vi "IECal-Compute ASTF.vi"(0 "Stimulus":dbl[](array[numeric]), 5 "Response":dbl[](array[numeric]), 7 "Fs (Hz)":dbl, 9 "Response":T1, 11 "error in (no error)":errorcluster) -> (6 "data":T2, 15 "error out":errorcluster)   [LabVIEW 2020]
uses:
  Common VIs/Typedefs/CAL-Data.ctl
  Typedefs/IECal-Response.ctl
  epl-vi-lib/Utility VIs/Math VIs/FFT x(t) to dB,Degrees (1D).vi
panel:
  out "Frequency":dbl[](array[numeric])
  out "ASTF Phase":dbl[](array[numeric])
  out "ASTF Mag":dbl[](array[numeric])
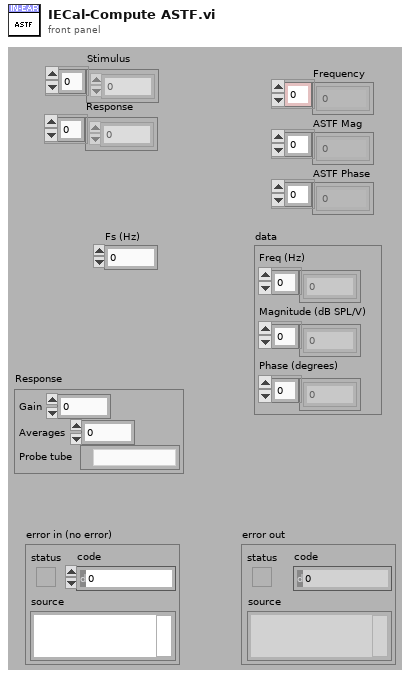
[diagram p1: front panel]
types:
  T1 = typedef "IECal-Response.ctl" = cluster{"Gain":dbl, "Averages":i32, "Probe tube":path}
  T2 = typedef "CAL-Data.ctl" = cluster{"Freq (Hz)":dbl[], "Magnitude (dB SPL/V)":dbl[], "Phase (degrees)":dbl[]}
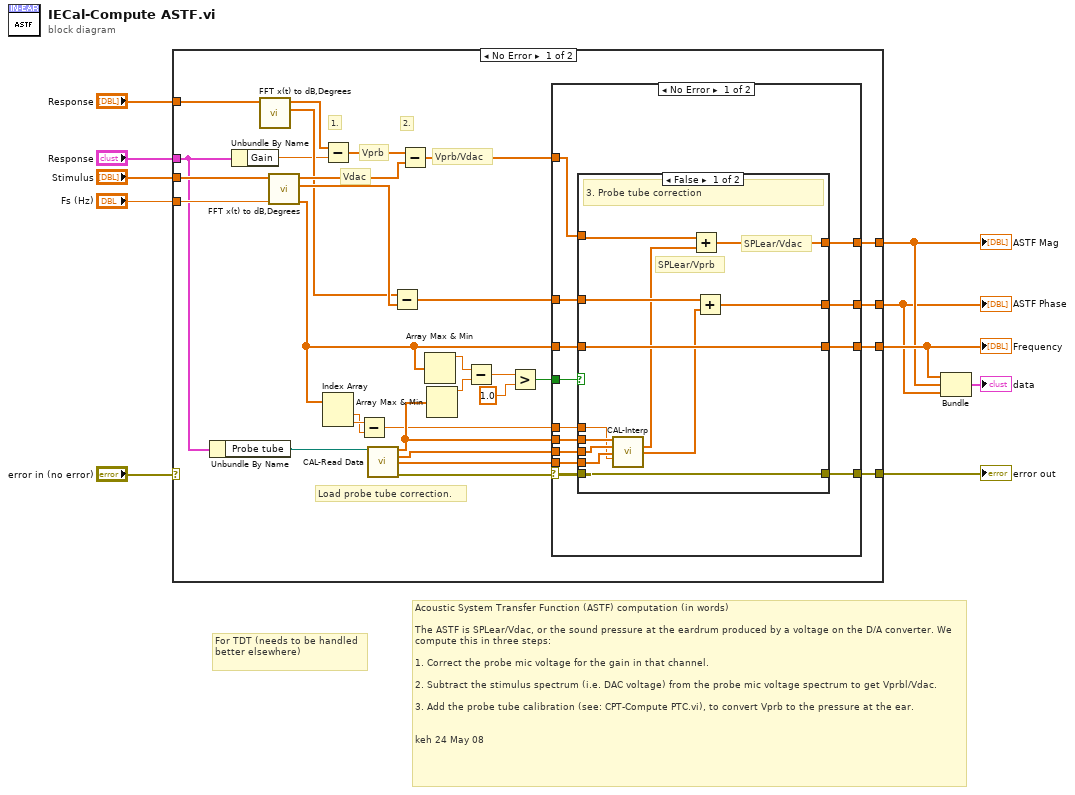
[diagram p0: block diagram]
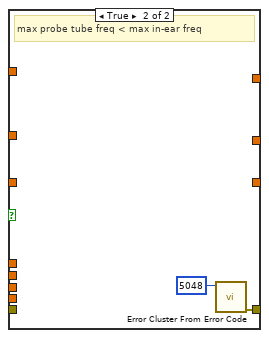
[diagram p2: hidden frame]
diagram:
  # "For TDT (needs to be handled better elsewhere)"
  # "Acoustic System Transfer Function (ASTF) computation (in words)\n\nThe ASTF is SPLear/Vdac, or the sound pressure at the eardrum produced by a voltage on the D/A converter. We compute this in three steps:\n\n1. Correct the probe mic voltage for the gain in that channel.\n\n2. Subtract the stimulus spectrum (i.e. DAC voltage) from the probe mic voltage spectrum to get Vprbl/Vdac.\n\n3. Add the probe tube calibration (see: CPT-Compute PTC.vi), to convert Vprb to the pressure at the ear.\n\n\nkeh 24 May 08"
  n1 = case shown="No Error" "error in (no error)" {
    selector: "error in (no error)" -> [_ w69]
    tunnel: "Response" -> [w21 _]
    tunnel: [w40 _] -> w4
    tunnel: [w39 _] -> w3
    tunnel: "Stimulus" -> [w33 _]
    tunnel: "Fs (Hz)" -> [w18 _]
    tunnel: [w28 _] -> w5
    tunnel: [w35 w69] -> w6
    tunnel: "Response" -> [w12 _]
    frame No Error {
      # "Load probe tube correction."
      # "2."
      # "1."
      # "Vprb/Vdac"
      # "Vdac"
      # "Vprb"
      n2 = Unbundle By Name(w12) -> ("Probe tube"=w11:path)
      n3 = Unbundle By Name(w12) -> ("Gain"=w13:dbl)
      n4 = call-poly "FFT x(t) to dB,Degrees.vi"("X"=w21) -> ("+Freq Phase of FFT (degrees)"=w19:dbl[], "+Freq. Mag of FFT (dB rms)"=w20:dbl[])  [unwired: 8 in, 1 out]
      n5 = call-poly "FFT x(t) to dB,Degrees.vi"("Fs (Hz)"=w18, "X"=w33) -> ("Freq (Hz)"=w17:dbl[], "+Freq Phase of FFT (degrees)"=w24:dbl[], "+Freq. Mag of FFT (dB rms)"=w32:dbl[])  [unwired: 7 in]
      n6 = Subtract(x=w20, y=w13) -> (x-y=w37:dbl[])
      n7 = Index Array(array=w17) -> (element #1=w15:dbl, element #2=w16:dbl)  [unwired: 2 in]
      n8 = Subtract(x=w16, y=w15) -> (x-y=w14:dbl)
      n9 = call "CAL-Read Data.vi"("user path"=w11) -> ("Frequency (Hz)"=w27:dbl[], "Mag"=w26:dbl[], "Phase"=w25:dbl[], "error out"=w36:errorcluster)  [unwired: 10 in, 1 out]
      n10 = Subtract(x=w19, y=w24) -> (x-y=w38:dbl[])
      n11 = Subtract(x=w37, y=w32) -> (x-y=w34:dbl[])
      n12 = Array Max & Min(array=w17) -> (max value=w31:dbl)  [unwired: 3 out]
      n13 = Array Max & Min(array=w27) -> (max value=w30:dbl)  [unwired: 3 out]
      n14 = Subtract(x=w31, y=w30) -> (x-y=w29:dbl)
      n15 = Greater?(x=w29, y=1.0) -> (0:w23:bool)
      n16 = case shown="No Error" w36 {
        selector: w36 -> [w50 w68]
        tunnel: [w41 _] -> w40
        tunnel: [w53 _] -> w39
        tunnel: w38 -> [w52 _]
        tunnel: w23 -> [w51 _]
        tunnel: w34 -> [w43 _]
        tunnel: [w42 w68] -> w35
        tunnel: w17 -> [w49 _]
        tunnel: [w44 _] -> w28
        tunnel: w14 -> [w48 _]
        tunnel: w27 -> [w47 _]
        tunnel: w26 -> [w46 _]
        tunnel: w25 -> [w45 _]
        frame No Error {
          n17 = case shown="False" w51 {
            tunnel: w43 -> [w55 _]
            tunnel: [w65 _] -> w53
            tunnel: w52 -> [w64 _]
            tunnel: [w63 w67] -> w42
            tunnel: w50 -> [w63 _]
            tunnel: w49 -> [w62 _]
            tunnel: [w62 _] -> w44
            tunnel: w48 -> [w58 _]
            tunnel: w47 -> [w61 _]
            tunnel: w46 -> [w60 _]
            tunnel: w45 -> [w59 _]
            tunnel: [w54 _] -> w41
            frame False {
              # "SPLear/Vprb"
              # "SPLear/Vdac"
              # "3. Probe tube correction"
              n18 = call "CAL-Interp.vi"("Frequency (Hz)"=w61, "Magnitude (dB)"=w60, "Phase (degrees)"=w59, "df (Hz)"=w58) -> ("Interp Magnitude (dB)"=w57:dbl[], "Interp Phase (degrees)"=w56:dbl[])  [unwired: 8 in, 2 out]
              n19 = Add(x=w55, y=w57) -> (x+y=w54:dbl[])
              n20 = Add(x=w64, y=w56) -> (x+y=w65:dbl[])
            }
            frame True {
              # "max probe tube freq < max in-ear freq"
              n21 = call <vilib>:"Error Cluster From Error Code.vi"("error code (0)"=5048) -> ("error out"=w67:errorcluster)  [unwired: 8 in]
            }
          }
        }
        frame Error {
        }
      }
    }
    frame Error {
    }
  }
  "ASTF Mag" <- w4
  "ASTF Phase" <- w3
  "error out" <- w6
  "Frequency" <- w5
  n22 = Bundle("Freq (Hz)"=w5, w4, w3) -> (→"data":cluster{"Freq (Hz)":dbl[], dbl[], dbl[]})  [unwired: 1 in]
